vi "Read Real.vi"(11 "GDSII.DataType.Real in":refnum<class "GDSII.DataType.Real.lvclass">) -> (2 "Real":dbl[](array[numeric]), 3 "GDSII.DataType.Real out":refnum<class "GDSII.DataType.Real.lvclass">)   [LabVIEW 2019, in "GDSII.DataType.Real.lvclass"]
uses:
  GDSII.DataType.Real.lvclass
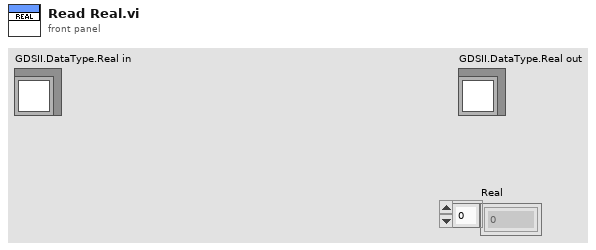
[diagram p1: front panel]
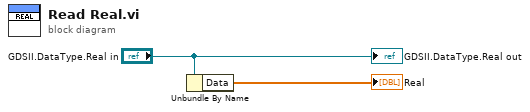
[diagram p0: block diagram]
diagram:
  n1 = Unbundle By Name("GDSII.DataType.Real in") -> ("Data"=→"Real":dbl[])
  "GDSII.DataType.Real out" <- "GDSII.DataType.Real in"
